vi "Mark_BE_Thrd.vi"(4 "Output Type":enum16{"Time", "Percentage", "Index"}(ring), 5 "End Time":dbl, 6 "threshold":dbl, 7 "Start Time":dbl, 8 "error in (no error)":errorcluster, 9 "Input":dbl[](array[numeric]), 10 "Time":dbl[](array[numeric]), 11 "CarexData In":refnum<class "ExpData.lvclass">) -> (0 "error out":errorcluster, 1 "End":dbl[](array[numeric]) format="%.2f", 2 "Begin":dbl[](array[numeric]) format="%.2f", 3 "CarexData Out":refnum<class "ExpData.lvclass">)   [LabVIEW 2015, in "ExpData.lvclass"]
uses:
  ExpData.lvclass
  <vilib>/Analysis/3filter.llb/Filter Passband Type.ctl
  ExpData.lvclass/ExpData.ctl
  <vilib>/Analysis/3filter.llb/Zero Phase Filter (Cascade, DBL).vi
  <userlib>/_OpenG.lib/array/array.llb/Conditional Auto-Indexing Tunnel (I32)__ogtk.vi
  <userlib>/_OpenG.lib/array/array.llb/Index 1D Array Elements (DBL)__ogtk.vi
  <vilib>/Analysis/NI_AALPro.lvlib
  <vilib>/Analysis/NI_AALBase.lvlib
panel:
  out "Before 2":dbl[](graph)
  out "After":dbl[](graph)
  out "Before":dbl[](graph)
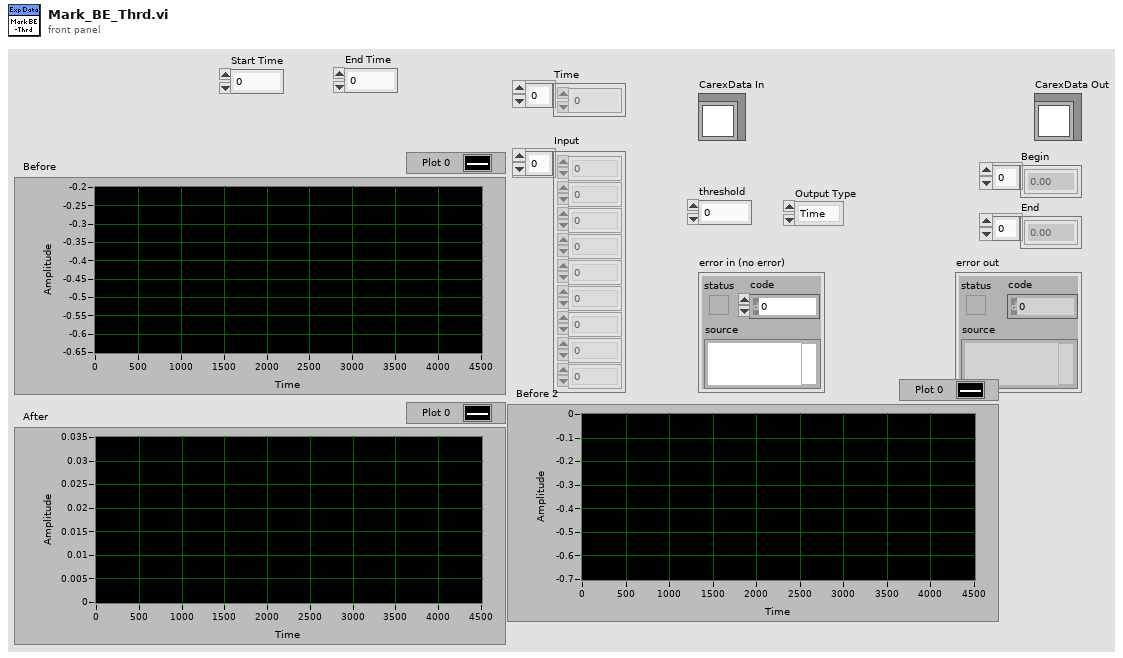
[diagram p1: front panel]
types:
  T1 = typedef "NI_AALBase.lvlib/Filter Passband Type.ctl" = enum32{"Lowpass", "Highpass", "Bandpass", "Bandstop"}
  T2 = cluster{"filter structure":enum32{"IIR 2nd Order", "IIR 4th Order"}, "Reverse Coefficients":dbl[], "Forward Coefficients":dbl[]}
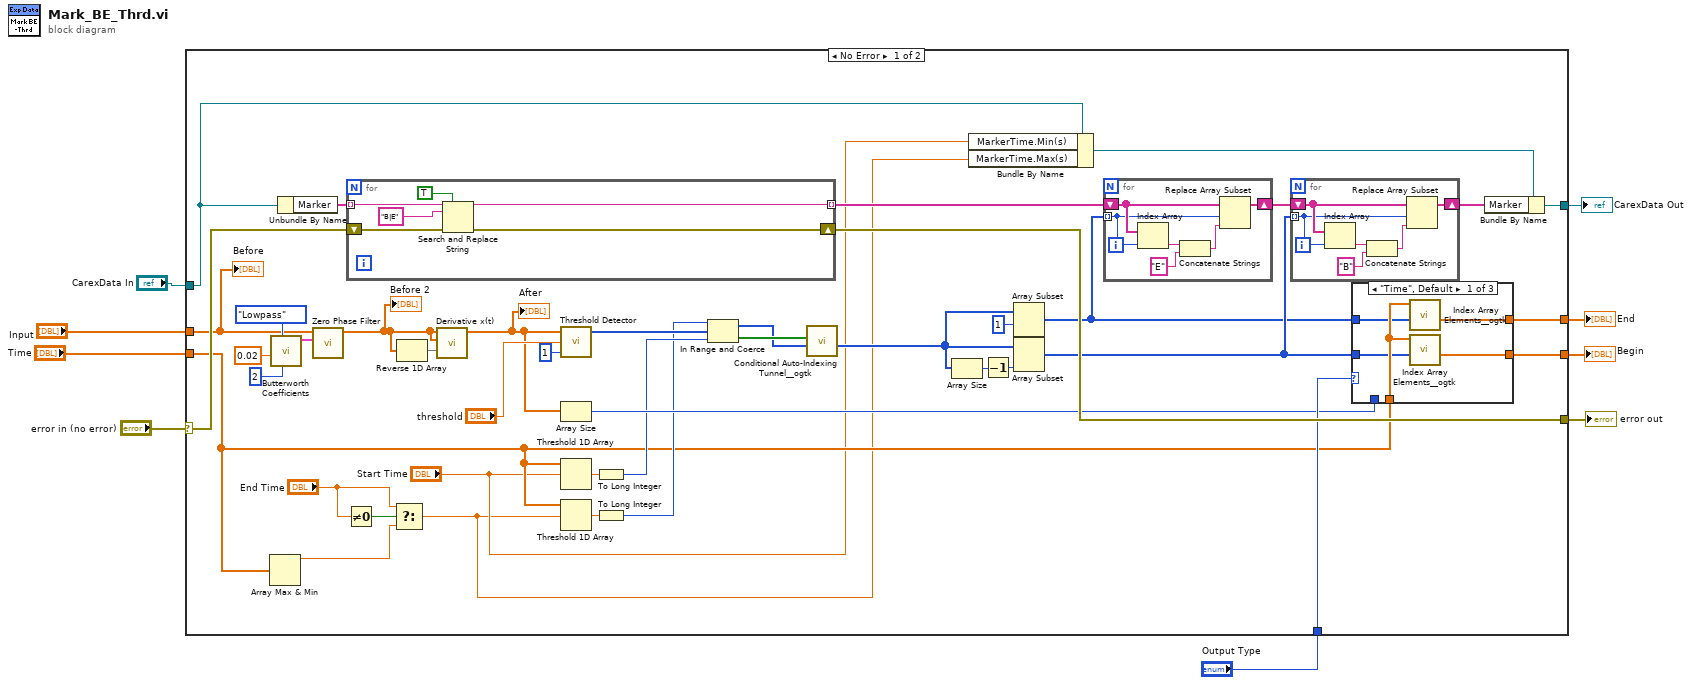
[diagram p0: block diagram]
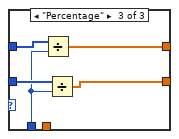
[diagram p3: hidden frame]
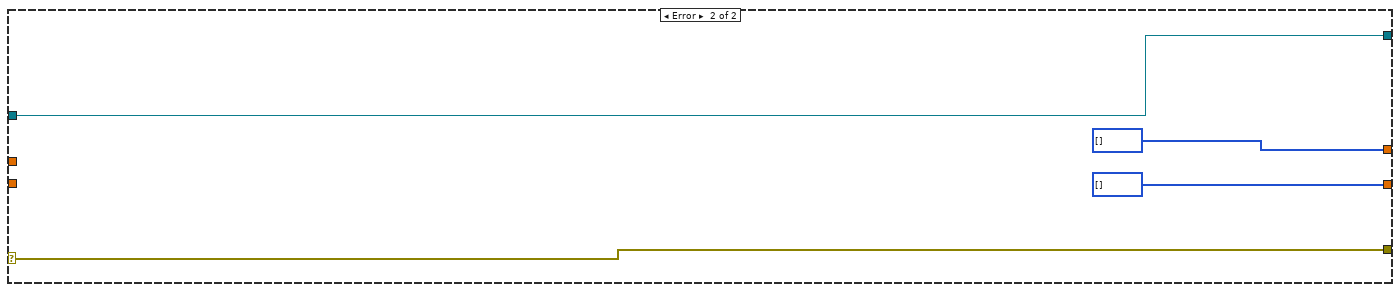
[diagram p4: hidden frame]
diagram:
  n1 = case shown="No Error" "error in (no error)" {
    selector: "error in (no error)" -> [w37 w85]
    tunnel: [w46 w85] -> w9
    tunnel: "CarexData In" -> [w13 w82]
    tunnel: [w41 i32[] []] -> w6
    tunnel: [w39 i32[] []] -> w5
    tunnel: [w44 w82] -> w4
    tunnel: "Output Type" -> [w38 _]
    tunnel: "Time" -> [w20 _]
    tunnel: "Input" -> [w32 _]
    frame No Error {
      n2 = Array Max & Min(array=w20) -> (max value=w19:dbl)  [unwired: 3 out]
      n3 = call <vilib>:"Butterworth Coefficients.vi"("order"=2, "filter type"=Filter_Passband_Type."Lowpass", "low cutoff freq: fl"=0.02 ("high cutoff freq: fh")) -> ("IIR Filter Cluster"=w34:T2)  [unwired: 7 in, 1 out]
      n4 = Unbundle By Name(w13) -> ("Marker"=w43:string[])
      n5 = call-poly <vilib>:"Zero Phase Filter.vi"("IIR Filter Cluster"=w34, "X"=w32) -> ("Filtered X"=w30:dbl[])  [unwired: 8 in, 1 out]
      "Before 2" <- w30
      n6 = Not Equal To 0?(x="End Time") -> (x != 0?=w18:bool)
      n7 = for {
        tunnel: w43 -> [w69] mode=indexing
        tunnel: [w67] -> w47 mode=indexing
        shift-right: [w64] -> w46
        shift-left: w37 -> [w65]
        n8 = Search and Replace String(replace all?=TRUE ("replace all? (F)"), input string=w69, search string="B|E", error in=w65) -> (result string=w67:string, error out=w64:errorcluster)  [unwired: 4 in, 2 out]
      }
      n9 = Select(t="End Time", s=w18, f=w19) -> (s? t:f=w10:dbl)
      n10 = Reverse 1D Array(array=w30) -> (reversed array=w31:dbl[])
      n11 = call <vilib>:"Derivative x(t).vi"("Final Condition"=w31, "Initial Condition"=w30, "X"=w30) -> ("dX/dt"=w26:dbl[])  [unwired: 7 in, 1 out]
      "After" <- w26
      n12 = call <vilib>:"Threshold Detector.vi"("width"=1, "threshold"="threshold", "X"=w26) -> ("Indices"=w25:i32[])  [unwired: 2 out]
      n13 = Array Size(array=w26) -> (size(s)=w27:i32)
      n14 = Threshold 1D Array(2:"Start Time", 3:w20) -> (0:w24:dbl)  [unwired: 1 in]
      n15 = Threshold 1D Array(2:w10, 3:w20) -> (0:w23:dbl)  [unwired: 1 in]
      n16 = To Long Integer(number=w24) -> (32bit integer=w22:i32)
      n17 = To Long Integer(number=w23) -> (32bit integer=w21:i32)
      n18 = In Range and Coerce(upper limit=w21, x=w25, lower limit=w22) -> (coerced(x)=w15:i32[], In Range?=w16:bool[])
      n19 = call-poly <userlib>:"Conditional Auto-Indexing Tunnel__ogtk.vi"("Array in"=w15, "Elements to keep"=w16) -> ("Filtered Array out"=w14:i32[])  [unwired: 5 in]
      n20 = Array Size(array=w14) -> (size(s)=w51:i32)
      n21 = Bundle By Name(cluster=w13, "MarkerTime.Min(s)"="Start Time", "MarkerTime.Max(s)"=w10) -> (w12:refnum<class "ExpData.lvclass">)
      n22 = Decrement(x=w51) -> (x-1=w50:i32)
      n23 = Array Subset(array=w14, index=1) -> (w40:i32[])  [unwired: 1 in]
      n24 = Array Subset(array=w14, length=w50) -> (w42:i32[])  [unwired: 1 in]
      n25 = for {
        tunnel: w40 -> [w79] mode=indexing
        shift-right: [w81] -> w48
        shift-left: w47 -> [w80]
        n26 = Index Array(array=w80, index=w79) -> (element=w77:string)
        n27 = Concatenate Strings(w77, "E" ("new element/subarray")) -> (w78:string)
        n28 = Replace Array Subset(array=w80, new element=w78, index=w79) -> (w81:string[])
      }
      n29 = for {
        tunnel: w42 -> [w73] mode=indexing
        shift-right: [w75] -> w45
        shift-left: w48 -> [w74]
        n30 = Index Array(array=w74, index=w73) -> (element=w71:string)
        n31 = Concatenate Strings(w71, "B" ("new element/subarray")) -> (w72:string)
        n32 = Replace Array Subset(array=w74, new element=w72, index=w73) -> (w75:string[])
      }
      n33 = case shown="\"Time\", Default" w38 {
        tunnel: w42 -> [w53 w58 w61]
        tunnel: [w52 w58 w59] -> w41
        tunnel: w40 -> [w55 w57 w63]
        tunnel: [w54 w57 w62] -> w39
        tunnel: w27 -> [_ _ w60]
        tunnel: w20 -> [w56 _ _]
        frame "Time", Default {
          n34 = call-poly <userlib>:"Index Array Elements__ogtk.vi"("indices"=w55, "array"=w56) -> ("elements"=w54:dbl[])  [unwired: 9 in]
          n35 = call-poly <userlib>:"Index Array Elements__ogtk.vi"("indices"=w53, "array"=w56) -> ("elements"=w52:dbl[])  [unwired: 9 in]
        }
        frame "Index" {
        }
        frame "Percentage" {
          n36 = Divide(x=w63, y=w60) -> (x/y=w62:dbl[])
          n37 = Divide(x=w61, y=w60) -> (x/y=w59:dbl[])
        }
      }
      n38 = Bundle By Name(cluster=w12, "Marker"=w45) -> (w44:refnum<class "ExpData.lvclass">)
      "Before" <- w32
    }
    frame Error {
    }
  }
  "CarexData Out" <- w4
  "error out" <- w9
  "Begin" <- w6
  "End" <- w5
